vi "Get Output.vi"(8 "error in (no error)":errorcluster, 11 "Modbus Master in":refnum<class "Modbus Master.lvclass">) -> (0 "error out":errorcluster, 2 "Temperature (C)":dbl, 3 "Modbus Master out":refnum<class "Modbus Master.lvclass">)   [LabVIEW 2023, in "PIDModbus.lvlib"]
uses:
  <vilib>/NI/Modbus Library/API/Master/Modbus Master.lvclass
  Controls/Register Enum.ctl
  PIDModbus.lvlib
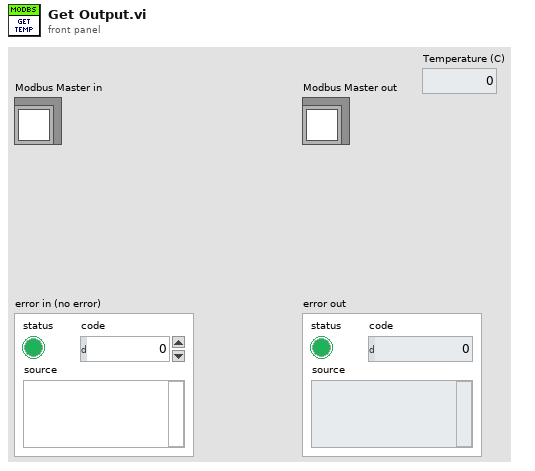
[diagram p1: front panel]
types:
  T1 = typedef "PIDModbus.lvlib/Register Enum.ctl" = u16
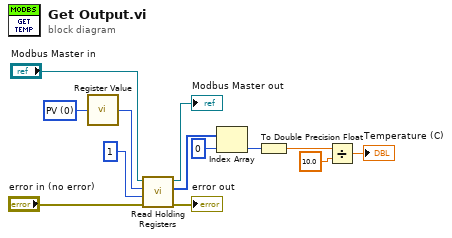
[diagram p0: block diagram]
diagram:
  w7 = T1 0 items=["PV"=0, "SV"=5, "P1"=24, "I1"=25, "D1"=26] ("Register")
  n1 = call "Register Value.vi"("Register"=w7) -> ("RegAddr (Hex)"=w6:u16)
  n2 = call-dynamic "Read Holding Registers.vi"("error in"="error in (no error)", "number of inputs"=u16 1, "starting address"=w6, "Modbus master in"="Modbus Master in") -> ("error out"=→"error out":errorcluster, "register values"=w11:u16[], "Modbus master out"=→"Modbus Master out":refnum<class "Modbus Master.lvclass">)  [unwired: 5 in]
  n3 = Index Array(array=w11, index=0) -> (element=w4:u16)
  n4 = To Double Precision Float(number=w4) -> (double precision float=w2:dbl)
  n5 = Divide(x=w2, y=10.0) -> (x/y=→"Temperature (C)":dbl)
